vi "Generate Test Images.vi"() -> (0 "error out":errorcluster, 1 "queue out":refnum<queue>)   [LabVIEW 2023]
doc: "Generate 50 test images of each type of board, with randomized failures."
uses:
  Assembly Line Input.ctl
  Board Image.ctl
  Board Type Enum.ctl
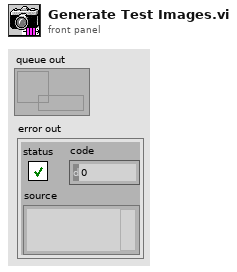
[diagram p1: front panel]
types:
  T1 = typedef "Assembly Line Input.ctl" = cluster{"board image":T2, "which board":T3}
  T2 = typedef "Board Image.ctl" = picture
  T3 = typedef "Board Type Enum.ctl" = enum16{"Basic DAQ Board", "Elite DAQ Board", "GPIB Board"}
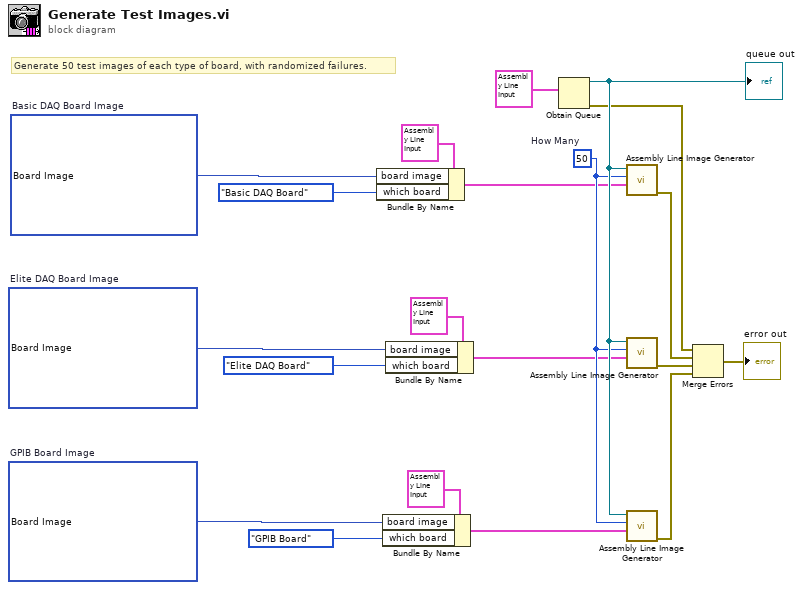
[diagram p0: block diagram]
diagram:
  w6 = T2 bytes[67710]  # GPIB Board Image
  w9 = T2 bytes[67710]  # Elite DAQ Board Image
  w11 = T2 bytes[67710]  # Basic DAQ Board Image
  w19 = 50  # How Many
  # "Generate 50 test images of each type of board, with randomized failures."
  n1 = Bundle By Name(cluster=T1 {"board image"=bytes[0], "which board"=enum."Basic DAQ Board"} ("Assembly Line Input"), "board image"=w11, "which board"=Board_Type_Enum."Basic DAQ Board") -> (w4:T1)
  n2 = Bundle By Name(cluster=T1 {"board image"=bytes[0], "which board"=enum."Basic DAQ Board"} ("Assembly Line Input"), "board image"=w6, "which board"=Board_Type_Enum."GPIB Board") -> (w2:T1)
  n3 = Bundle By Name(cluster=T1 {"board image"=bytes[0], "which board"=enum."Basic DAQ Board"} ("Assembly Line Input"), "board image"=w9, "which board"=Board_Type_Enum."Elite DAQ Board") -> (w3:T1)
  n4 = Obtain Queue(element data type=T1 {"board image"=bytes[0], "which board"=enum."Basic DAQ Board"} ("Assembly Line Input")) -> (queue out=w20:refnum<queue>, error out=w14:errorcluster)  [unwired: 4 in, 1 out]
  "queue out" <- w20
  n5 = call "Assembly Line Image Generator.vi"("assembly line input"=w4, "how many"=w19, "Queue in"=w20) -> ("error out"=w18:errorcluster)  [unwired: 8 in]
  n6 = call "Assembly Line Image Generator.vi"("assembly line input"=w3, "how many"=w19, "Queue in"=w20) -> ("error out"=w17:errorcluster)  [unwired: 8 in]
  n7 = call "Assembly Line Image Generator.vi"("assembly line input"=w2, "how many"=w19, "Queue in"=w20) -> ("error out"=w16:errorcluster)  [unwired: 8 in]
  n8 = Merge Errors(w14, w18, w17, w16) -> (→"error out":errorcluster)
